vi "New Go.vi"() -> ()   [LabVIEW 2020]
uses:
  Aerotech.lvlib
  Program Files (x86)/Aerotech/A3200/LabVIEW/2010/Motion/WaitSingle.vi
  Controller/Dispenser/Dispenser.lvclass
  Program Files (x86)/Aerotech/A3200/LabVIEW/2010/Motion/MoveIncSingle.vi
  Program Files (x86)/Aerotech/A3200/LabVIEW/2010/Motion/WaitMultiple.vi
  Controller/Motion/Motion.lvclass
  CAD Dispense/CAD Dispense.lvclass
  C:/Users/hep/Documents/CMU gantry/Classes/Routine/Dispense/Dispense.lvclass
  C:/Users/hep/Documents/CMU gantry/Classes/Routine/Routine.lvclass
  C:/Users/hep/Documents/CMU gantry/Classes/Routine/Dispense/CAD Dispense/CAD Dispense.lvclass
  Controller/I-O/I-O.lvclass
  Controller/Controllers.ctl
  Controller/Controller.lvclass
  C:/Program Files (x86)/Aerotech/A3200/LabVIEW/2010/Bin/Aerotech.A3200.dll
  Program Files (x86)/Aerotech/A3200/LabVIEW/2010/Bin/Aerotech.A3200.dll
panel:
  out "Control Out":T1
  in  "Control In":T1
  out "CAD Dispense Out":refnum<class "CAD Dispense.lvclass">
  in  "CAD Dispense in":refnum<class "CAD Dispense.lvclass">
  in  "Timing Values":dbl[](array[numeric])
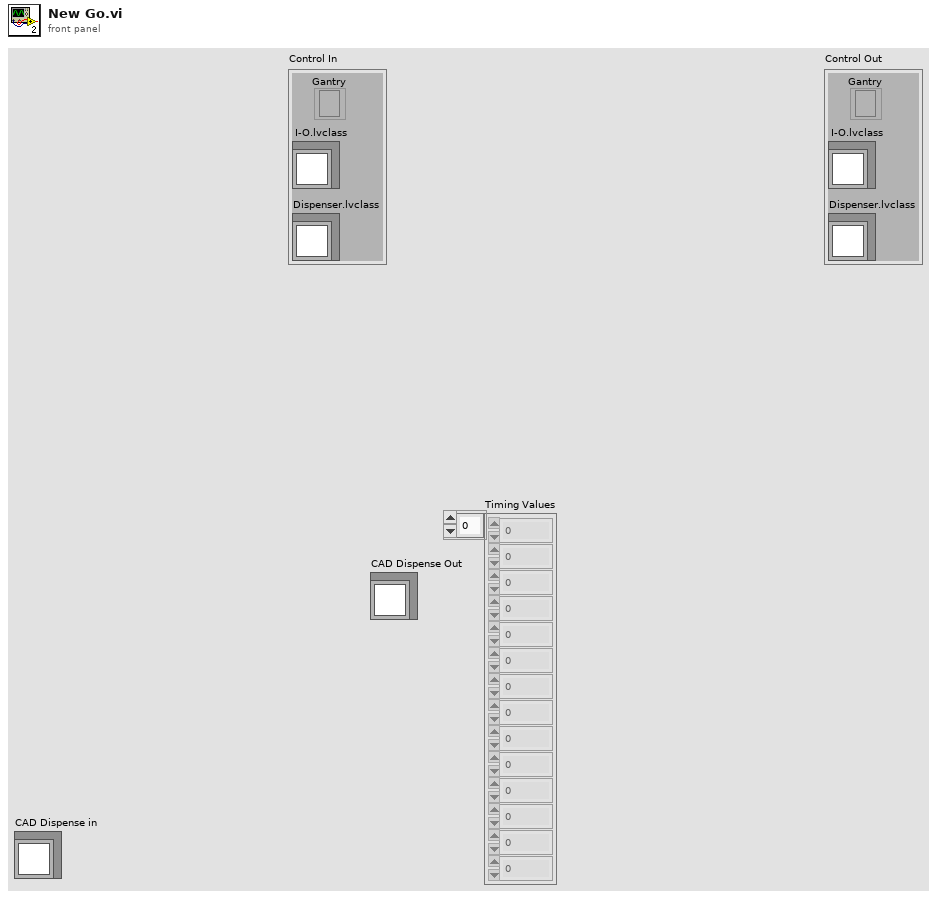
[diagram p1: front panel]
types:
  T1 = typedef "Controller.lvclass/Controllers.ctl" = cluster{"I-O.lvclass":refnum<class "I-O.lvclass">, "Dispenser.lvclass":refnum<class "Dispenser.lvclass">, "Gantry":refnum<k24>}
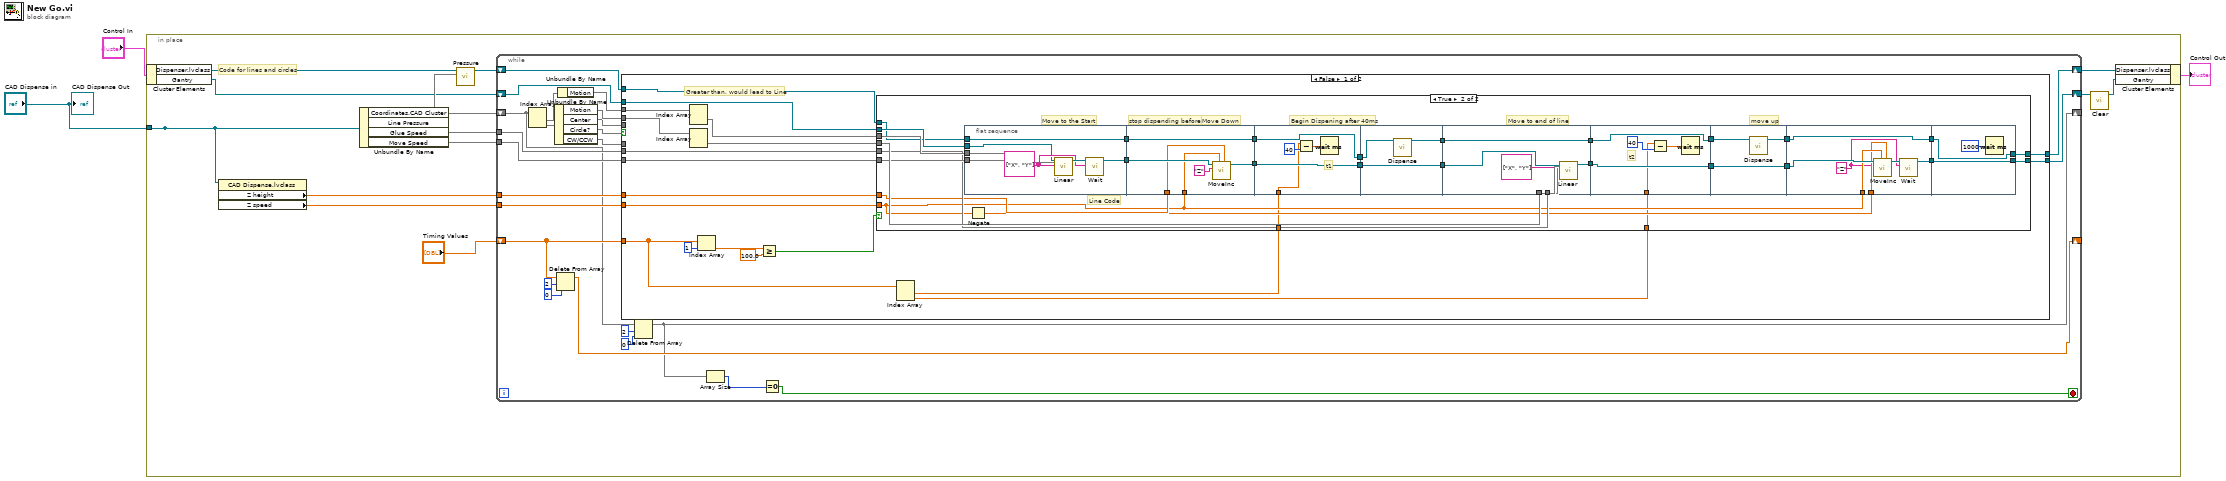
[diagram p0: block diagram]
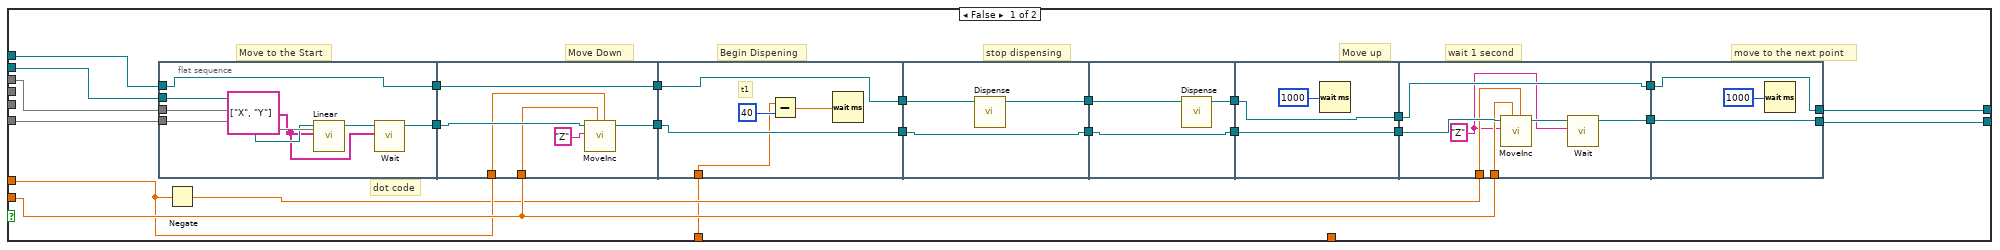
[diagram p2: hidden frame]
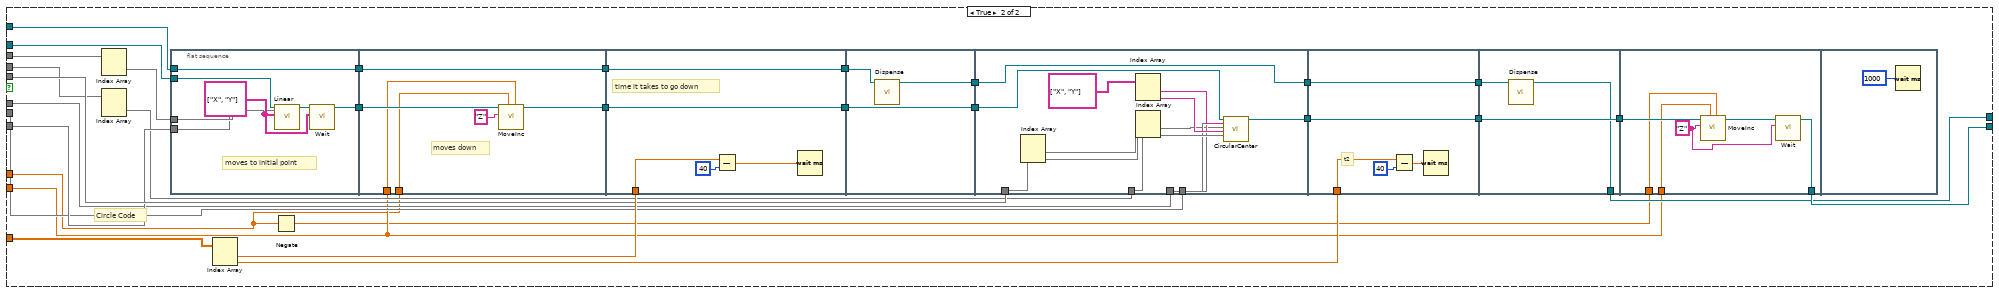
[diagram p3: hidden frame]
diagram:
  n1 = in-place {
    in-place-border: "CAD Dispense in" -> [w4]
    # "Code for lines and circles"
    n2 = in-place-cluster #1("Control In") -> ("Dispenser.lvclass"=w7:refnum<class "Dispenser.lvclass">, "Gantry"=w8:refnum<k24>)
    n3 = property class="CAD Dispense.lvclass"(reference=w4) -> ("Z height"=w11:dbl, "Z speed"=w12:dbl)  [unwired: 1 in, 2 out]
    n4 = Unbundle By Name "Unbundle By Name"(w4) -> ("Coordinates.CAD Cluster"=w15, "Line Pressure"=w14, "Glue Speed"=w10, "Move Speed"=w17)
    n5 = call-dynamic "Pressure.vi"("Pressure"=w14, "Dispenser in"=w7) -> ("Dispenser out"=w13:refnum<class "Dispenser.lvclass">)  [unwired: 8 in, 1 out]
    n6 = while {
      shift-right: [w34] -> w5
      shift-left: w13 -> [w35]
      tunnel: w17 -> [w39]
      shift-right: [w36] -> w9
      shift-left: w8 -> [w40]
      shift-right: [w24] -> _
      shift-left: "Timing Values" -> [w25]
      shift-right: [w20] -> _
      shift-left: w15 -> [w21]
      tunnel: w12 -> [w33]
      tunnel: w11 -> [w32]
      tunnel: w10 -> [w31]
      stop <- w18 stop-if-true
      n7 = Index Array(array=w21) -> (element #1=w42, element #2=w38)  [unwired: 2 in]
      n8 = Unbundle By Name(w38) -> ("Motion"=w37, "Center"=w29, "Circle?"=w30, "CW/CCW"=w28)
      n9 = Delete From Array(array=w25, length=2, index=0) -> (array with subset deleted=w24:dbl[])  [unwired: 1 out]
      n10 = Unbundle By Name(w42) -> ("Motion"=w41)
      n11 = case shown="False" w30 {
        tunnel: w25 -> [w45 w213]
        tunnel: w29 -> [_ w225]
        tunnel: w41 -> [w57 w224]
        tunnel: w40 -> [w53 w223]
        tunnel: w39 -> [w49 w222]
        tunnel: w37 -> [w54 w201]
        tunnel: [w52 w214] -> w36
        tunnel: w35 -> [w51 w212]
        tunnel: [w50 w205] -> w34
        tunnel: w33 -> [w47 w199]
        tunnel: w32 -> [w48 w198]
        tunnel: w31 -> [w46 w203]
        tunnel: w28 -> [_ w202]
        frame False {
          # "Greater than, would lead to Line"
          n12 = Index Array(array=w57) -> (element=w56)  [unwired: 2 in]
          n13 = Index Array(array=w54) -> (element=w55)  [unwired: 2 in]
          n14 = Index Array(array=w45, index=1) -> (element=w60:dbl)
          n15 = Greater Or Equal?(x=w60, y=100.0) -> (x >= y?=w58:bool)
          n16 = Index Array(array=w45) -> (element #1=w44:dbl, element #2=w43:dbl)  [unwired: 2 in]
          n17 = case shown="True" w58 {
            tunnel: w56 -> [w63 w151]
            tunnel: w55 -> [_ w150]
            tunnel: w53 -> [w85 w149]
            tunnel: [w77 w140] -> w52
            tunnel: w51 -> [w76 w139]
            tunnel: [w68 w130] -> w50
            tunnel: w49 -> [w67 w129]
            tunnel: w48 -> [w65 w127]
            tunnel: w47 -> [w66 w126]
            tunnel: w46 -> [_ w128]
            tunnel: w44 -> [w62 w124]
            tunnel: w43 -> [_ w123]
            frame False {
              # "dot code"
              # "stop dispensing"
              # "move to the next point"
              # "wait 1 second"
              # "Move up"
              # "Begin Dispening"
              # "Move Down"
              # "Move to the Start"
              n18 = flat-sequence {
                tunnel: w85 -> [w89]
                tunnel: [w92] -> w84
                tunnel: w76 -> [w91]
                tunnel: [w91] -> w73
                tunnel: w67 -> [w87]
                tunnel: w63 -> [w90]
                tunnel: w84 -> [w98]
                tunnel: [w97] -> w83
                tunnel: [w96] -> w74
                tunnel: w73 -> [w96]
                tunnel: w65 -> [w95]
                tunnel: w66 -> [w94]
                tunnel: w83 -> [w101]
                tunnel: [w101] -> w82
                tunnel: [w100] -> w75
                tunnel: w74 -> [w100]
                tunnel: w62 -> [w99]
                tunnel: w82 -> [w106]
                tunnel: [w106] -> w79
                tunnel: w75 -> [w105]
                tunnel: [w104] -> w72
                tunnel: [w109] -> w80
                tunnel: w79 -> [w109]
                tunnel: w72 -> [w108]
                tunnel: [w107] -> w69
                tunnel: [w111] -> w81
                tunnel: w80 -> [w111]
                tunnel: [w110] -> w70
                tunnel: w69 -> [w110]
                tunnel: w81 -> [w118]
                tunnel: [w117] -> w78
                tunnel: [w116] -> w71
                tunnel: w70 -> [w116]
                tunnel: w66 -> [w115]
                tunnel: w64 -> [w114]
                tunnel: w78 -> [w121]
                tunnel: [w121] -> w77
                tunnel: [w120] -> w68
                tunnel: w71 -> [w120]
                frame #0 {
                  w86 = string[] ["X", "Y"] ("axis names")
                  n19 = call "Linear.vi"("distances"=w90, "speed"=w87, "axis names"=w86, "controller in"=w89) -> ("controller out"=w88:refnum<k24>)  [unwired: 6 in, 1 out]
                  n20 = call-poly "Wait.vi"("axis names"=w86, "controller in"=w88) -> ("controller out"=w92:refnum<k24>)  [unwired: 7 in, 2 out]
                }
                frame #1 {
                  n21 = call-poly "MoveInc.vi"("distance"=w95, "speed"=w94, "axis name"="Z", "controller in"=w98) -> ("controller out"=w97:refnum<k24>)  [unwired: 6 in, 1 out]
                }
                frame #2 {
                  # "t1"
                  n22 = Subtract(x=w99, y=u32 40 ("milliseconds to wait")) -> (x-y=w102:dbl)
                  n23 = Wait (ms)(milliseconds to wait=w102) -> ()  [unwired: 1 out]
                }
                frame #3 {
                  n24 = call-dynamic "Dispense.vi"("Dispenser in"=w105) -> ("Dispenser out"=w104:refnum<class "Dispenser.lvclass">)  [unwired: 9 in, 1 out]
                }
                frame #4 {
                  n25 = call-dynamic "Dispense.vi"("Dispenser in"=w108) -> ("Dispenser out"=w107:refnum<class "Dispenser.lvclass">)  [unwired: 9 in, 1 out]
                }
                frame #5 {
                  n26 = Wait (ms)(milliseconds to wait=u32 1000) -> ()  [unwired: 1 out]
                }
                frame #6 {
                  w113 = "Z" ("axis name")
                  n27 = call-poly "MoveInc.vi"("distance"=w114, "speed"=w115, "axis name"=w113, "controller in"=w118) -> ("controller out"=w119:refnum<k24>)  [unwired: 6 in, 1 out]
                  n28 = call-poly "Wait.vi"("axis name"=w113, "controller in"=w119) -> ("controller out"=w117:refnum<k24>)  [unwired: 7 in, 2 out]
                }
                frame #7 {
                  n29 = Wait (ms)(milliseconds to wait=u32 1000) -> ()  [unwired: 1 out]
                }
              }
              n30 = Negate(x=w65) -> (-x=w64:dbl)
            }
            frame True {
              # "Move to end of line"
              # "move up"
              # "stop dispending before 40ms"
              # "Begin Dispening after 40ms"
              # "Move Down"
              # "Move to the Start"
              # "Line Code"
              n31 = flat-sequence {
                tunnel: w151 -> [w155]
                tunnel: w149 -> [w152]
                tunnel: [w158] -> w148
                tunnel: w139 -> [w157]
                tunnel: [w157] -> w138
                tunnel: w129 -> [w156]
                tunnel: w148 -> [w164]
                tunnel: [w163] -> w147
                tunnel: w138 -> [w162]
                tunnel: [w162] -> w137
                tunnel: w127 -> [w161]
                tunnel: w126 -> [w160]
                tunnel: w147 -> [w167]
                tunnel: [w167] -> w146
                tunnel: w137 -> [w166]
                tunnel: [w166] -> w136
                tunnel: w124 -> [w165]
                tunnel: w146 -> [w172]
                tunnel: [w172] -> w145
                tunnel: w136 -> [w171]
                tunnel: [w170] -> w135
                tunnel: w150 -> [w176]
                tunnel: w145 -> [w173]
                tunnel: [w177] -> w144
                tunnel: w135 -> [w178]
                tunnel: [w178] -> w134
                tunnel: w128 -> [w175]
                tunnel: w144 -> [w181]
                tunnel: [w181] -> w143
                tunnel: w134 -> [w180]
                tunnel: [w180] -> w133
                tunnel: w123 -> [w179]
                tunnel: w143 -> [w186]
                tunnel: [w186] -> w142
                tunnel: w133 -> [w185]
                tunnel: [w184] -> w132
                tunnel: w142 -> [w193]
                tunnel: [w191] -> w141
                tunnel: w132 -> [w190]
                tunnel: [w190] -> w131
                tunnel: w126 -> [w189]
                tunnel: w125 -> [w188]
                tunnel: w141 -> [w195]
                tunnel: [w195] -> w140
                tunnel: w131 -> [w194]
                tunnel: [w194] -> w130
                frame #0 {
                  w153 = string[] ["X", "Y"] ("axis names")
                  n32 = call "Linear.vi"("distances"=w155, "speed"=w156, "axis names"=w153, "controller in"=w152) -> ("controller out"=w154:refnum<k24>)  [unwired: 6 in, 1 out]
                  n33 = call-poly "Wait.vi"("axis names"=w153, "controller in"=w154) -> ("controller out"=w158:refnum<k24>)  [unwired: 7 in, 2 out]
                }
                frame #1 {
                  n34 = call-poly "MoveInc.vi"("distance"=w161, "speed"=w160, "axis name"="Z", "controller in"=w164) -> ("controller out"=w163:refnum<k24>)  [unwired: 6 in, 1 out]
                }
                frame #2 {
                  # "t1"
                  n35 = Subtract(x=w165, y=u32 40 ("milliseconds to wait")) -> (x-y=w168:dbl)
                  n36 = Wait (ms)(milliseconds to wait=w168) -> ()  [unwired: 1 out]
                }
                frame #3 {
                  n37 = call-dynamic "Dispense.vi"("Dispenser in"=w171) -> ("Dispenser out"=w170:refnum<class "Dispenser.lvclass">)  [unwired: 9 in, 1 out]
                }
                frame #4 {
                  n38 = call "Linear.vi"("distances"=w176, "speed"=w175, "axis names"=string[] ["X", "Y"], "controller in"=w173) -> ("controller out"=w177:refnum<k24>)  [unwired: 6 in, 1 out]
                }
                frame #5 {
                  # "t2"
                  n39 = Subtract(x=w179, y=40) -> (x-y=w182:dbl)
                  n40 = Wait (ms)(milliseconds to wait=w182) -> ()  [unwired: 1 out]
                }
                frame #6 {
                  n41 = call-dynamic "Dispense.vi"("Dispenser in"=w185) -> ("Dispenser out"=w184:refnum<class "Dispenser.lvclass">)  [unwired: 9 in, 1 out]
                }
                frame #7 {
                  w187 = "Z" ("axis name")
                  n42 = call-poly "MoveInc.vi"("distance"=w188, "speed"=w189, "axis name"=w187, "controller in"=w193) -> ("controller out"=w192:refnum<k24>)  [unwired: 6 in, 1 out]
                  n43 = call-poly "Wait.vi"("axis name"=w187, "controller in"=w192) -> ("controller out"=w191:refnum<k24>)  [unwired: 7 in, 2 out]
                }
                frame #8 {
                  n44 = Wait (ms)(milliseconds to wait=u32 1000) -> ()  [unwired: 1 out]
                }
              }
              n45 = Negate(x=w126) -> (-x=w125:dbl)
            }
          }
        }
        frame True {
          # "Circle Code"
          n46 = Index Array(array=w224) -> (element=w204)  [unwired: 2 in]
          n47 = Index Array(array=w201) -> (element=w200)  [unwired: 2 in]
          n48 = flat-sequence {
            tunnel: w223 -> [w232]
            tunnel: w222 -> [w228]
            tunnel: [w234] -> w221
            tunnel: w212 -> [w233]
            tunnel: [w233] -> w209
            tunnel: w204 -> [w229]
            tunnel: w221 -> [w240]
            tunnel: [w239] -> w220
            tunnel: [w238] -> w210
            tunnel: w209 -> [w238]
            tunnel: w199 -> [w236]
            tunnel: w198 -> [w235]
            tunnel: w227 -> [w245]
            tunnel: w220 -> [w242]
            tunnel: [w242] -> w218
            tunnel: [w241] -> w211
            tunnel: w210 -> [w241]
            tunnel: [w248] -> w219
            tunnel: w218 -> [w248]
            tunnel: w211 -> [w247]
            tunnel: [w246] -> w206
            tunnel: w225 -> [w259]
            tunnel: w219 -> [w256]
            tunnel: [w255] -> w217
            tunnel: [w254] -> w207
            tunnel: w206 -> [w254]
            tunnel: w203 -> [w253]
            tunnel: w202 -> [w252]
            tunnel: w200 -> [w251]
            tunnel: w226 -> [w263]
            tunnel: w217 -> [w265]
            tunnel: [w265] -> w216
            tunnel: [w264] -> w208
            tunnel: w207 -> [w264]
            tunnel: w216 -> [w270]
            tunnel: [w270] -> w215
            tunnel: w208 -> [w269]
            tunnel: [w268] -> w205
            tunnel: w215 -> [w276]
            tunnel: [w274] -> w214
            tunnel: w199 -> [w273]
            tunnel: w197 -> [w272]
            frame #0 {
              w230 = string[] ["X", "Y"] ("axis names")
              # "moves to initial point"
              n49 = call "Linear.vi"("distances"=w229, "speed"=w228, "axis names"=w230, "controller in"=w232) -> ("controller out"=w231:refnum<k24>)  [unwired: 6 in, 1 out]
              n50 = call-poly "Wait.vi"("axis names"=w230, "controller in"=w231) -> ("controller out"=w234:refnum<k24>)  [unwired: 7 in, 2 out]
            }
            frame #1 {
              # "moves down"
              n51 = call-poly "MoveInc.vi"("distance"=w236, "speed"=w235, "axis name"="Z", "controller in"=w240) -> ("controller out"=w239:refnum<k24>)  [unwired: 6 in, 1 out]
            }
            frame #2 {
              # "time it takes to go down"
              n52 = Subtract(x=w245, y=u32 40 ("milliseconds to wait")) -> (x-y=w243:dbl)
              n53 = Wait (ms)(milliseconds to wait=w243) -> ()  [unwired: 1 out]
            }
            frame #3 {
              n54 = call-dynamic "Dispense.vi"("Dispenser in"=w247) -> ("Dispenser out"=w246:refnum<class "Dispenser.lvclass">)  [unwired: 9 in, 1 out]
            }
            frame #4 {
              n55 = Index Array "Index Array"(array=w259) -> (element #1=w258, element #2=w257)  [unwired: 2 in]
              n56 = Index Array(array=string[] ["X", "Y"]) -> (element #1=w262:string, element #2=w261:string)  [unwired: 2 in]
              n57 = Index Array(array=w251) -> (element #1=w250, element #2=w249)  [unwired: 2 in]
              n58 = call "CircularCenter.vi"("controller in"=w256, "axis 1 name"=w262, "axis 1 endpoint"=w250, "axis 2 name"=w261, "axis 2 endpoint"=w249, "speed"=w253, "axis 1 center point"=w258, "direction"=w252, "axis 2 center point"=w257) -> ("controller out"=w255:refnum<k24>)  [unwired: 9 in, 1 out]
            }
            frame #5 {
              # "t2"
              n59 = Subtract(x=w263, y=40) -> (x-y=w266:dbl)
              n60 = Wait (ms)(milliseconds to wait=w266) -> ()  [unwired: 1 out]
            }
            frame #6 {
              n61 = call-dynamic "Dispense.vi"("Dispenser in"=w269) -> ("Dispenser out"=w268:refnum<class "Dispenser.lvclass">)  [unwired: 9 in, 1 out]
            }
            frame #7 {
              w271 = "Z" ("axis name")
              n62 = call-poly "MoveInc.vi"("distance"=w272, "speed"=w273, "axis name"=w271, "controller in"=w276) -> ("controller out"=w275:refnum<k24>)  [unwired: 6 in, 1 out]
              n63 = call-poly "Wait.vi"("axis name"=w271, "controller in"=w275) -> ("controller out"=w274:refnum<k24>)  [unwired: 7 in, 2 out]
            }
            frame #8 {
              n64 = Wait (ms)(milliseconds to wait=u32 1000) -> ()  [unwired: 1 out]
            }
          }
          n65 = Index Array(array=w213) -> (element #1=w227:dbl, element #2=w226:dbl)  [unwired: 2 in]
          n66 = Negate(x=w198) -> (-x=w197:dbl)
        }
      }
      n67 = Delete From Array(array=w21, length=2, index=0) -> (array with subset deleted=w20)  [unwired: 1 out]
      n68 = Array Size(array=w20) -> (size(s)=w19:i32)
      n69 = Equal To 0?(x=w19) -> (x = 0?=w18:bool)
    }
    n70 = call "Clear.vi"("Gantry 2"=w9) -> ("Gantry 3"=w6:refnum<k24>)  [unwired: 9 in, 1 out]
    n71 = in-place-cluster #1("Dispenser.lvclass"=w5, "Gantry"=w6) -> (→"Control Out":T1)
  }
  "CAD Dispense Out" <- "CAD Dispense in"
